vi "Configure FP for custom mode.vi"(0 "reference in":refnum<class "SPWB.lvclass">, 5 "error in (no error)":errorcluster, 7 "Analysis Type":T1) -> (14 "reference out":refnum<class "SPWB.lvclass">, 19 "error out":errorcluster)   [LabVIEW 2022 SP3, in "SPWB.lvclass"]
uses:
  SPWB.lvclass
  controls/Analysis Type.ctl
panel:
  out "Control Labels":string[](array[string])
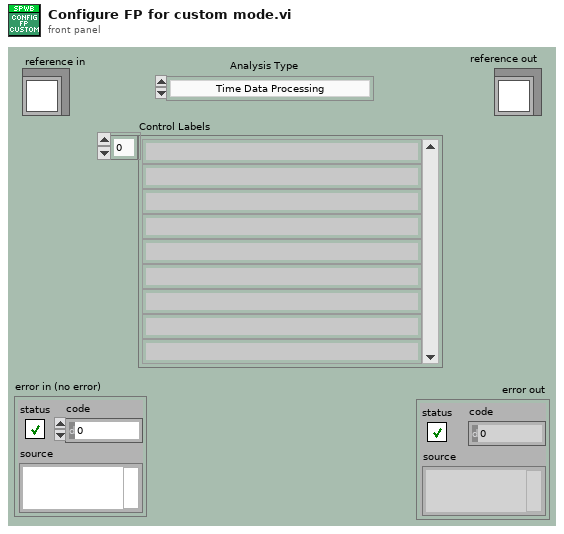
[diagram p1: front panel]
types:
  T1 = typedef "SPWB.lvclass/Analysis Type.ctl" = enum16{"Time Data Processing", "FFT Analysis", "Time Frequency Analysis", "Transfer Functions"}
  T2 = typedef "Generic Utilities.lvclass/FP Refnums.ctl" = cluster{"Panel refnum":refnum<vi>, "Control Labels":string[], "Refnums":refnum<vi>[]}
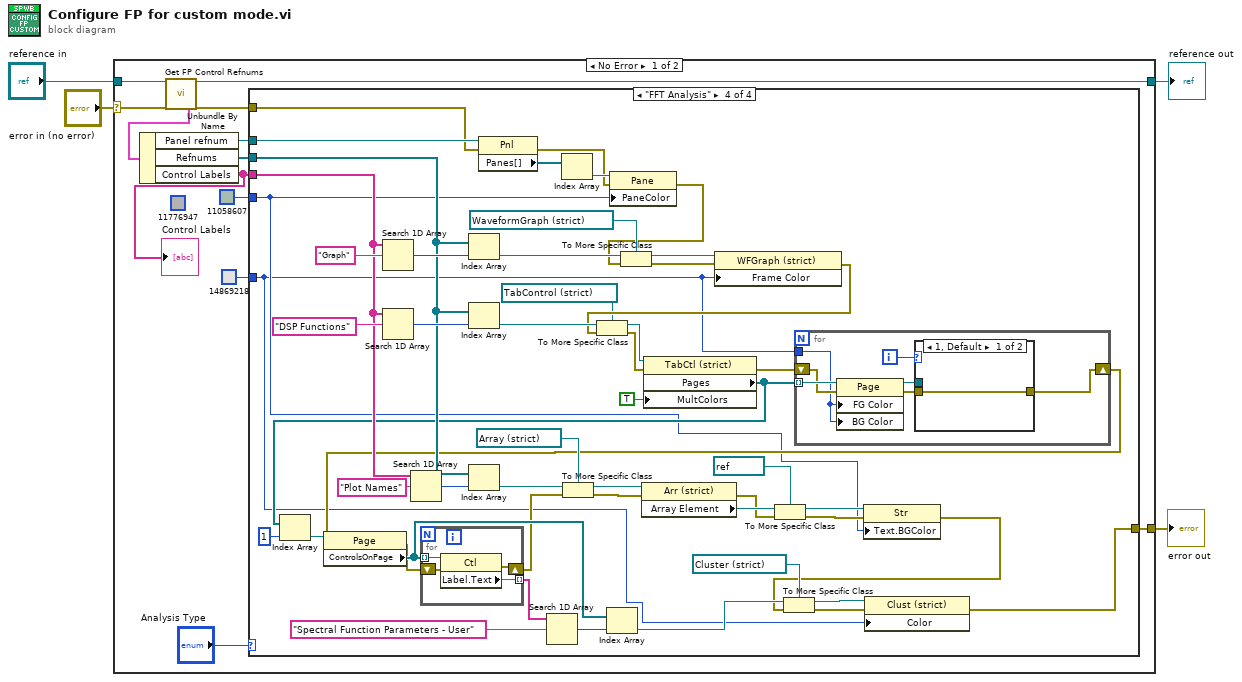
[diagram p0: block diagram]
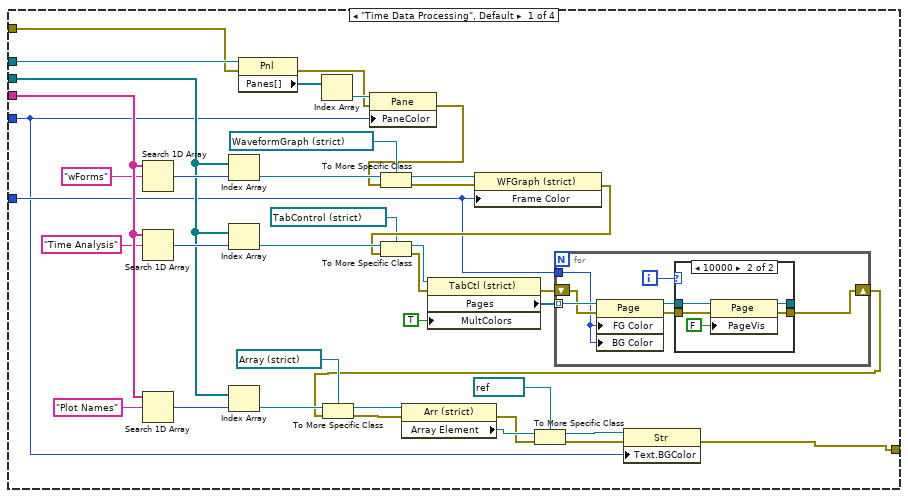
[diagram p2: hidden frame]
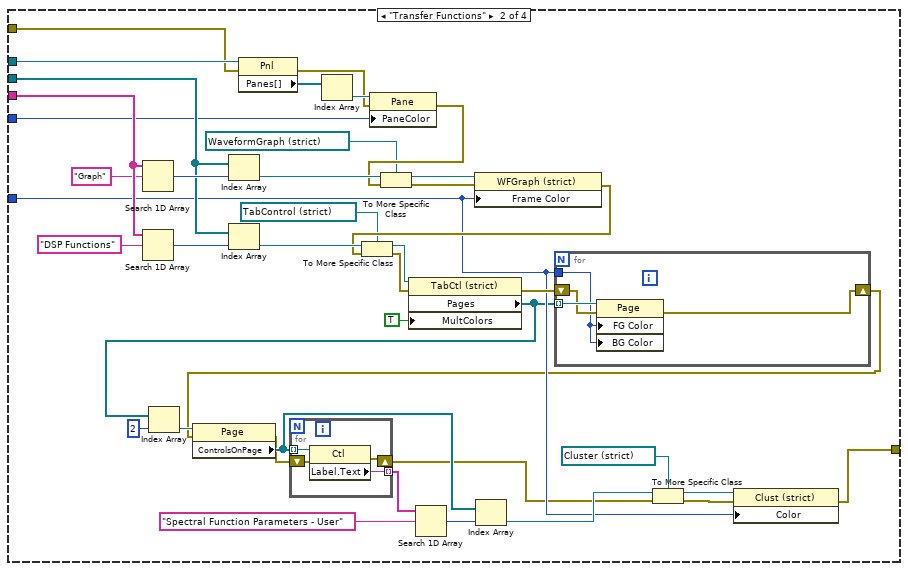
[diagram p4: hidden frame]
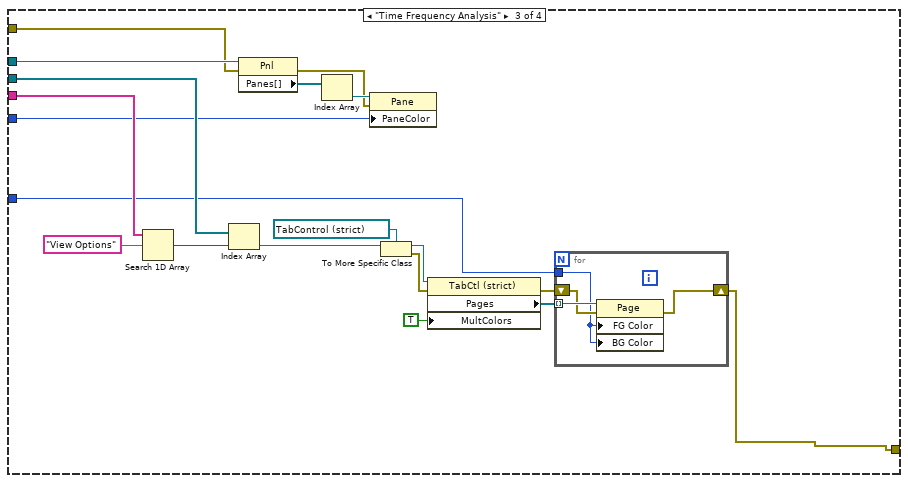
[diagram p5: hidden frame]
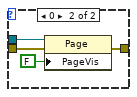
[diagram p6: hidden frame]
diagram:
  n1 = case shown="No Error" "error in (no error)" {
    selector: "error in (no error)" -> [w15 w210]
    tunnel: [w8 w210] -> w3
    tunnel: [w14 w209] -> w1
    tunnel: "reference in" -> [w16 w209]
    frame No Error {
      (unwired) u32 11776947
      n2 = call-dynamic "Get FP Control Refnums.vi"("reference in"=w16, "error in (no error)"=w15) -> ("FP Refnums"=w12:T2, "reference out"=w14:refnum<class "SPWB.lvclass">, "error out"=w9:errorcluster)  [unwired: 15 in]
      n3 = Unbundle By Name(w12) -> ("Panel refnum"=w10:refnum<vi>, "Refnums"=w11:refnum<vi>[], "Control Labels"=w7:string[])
      "Control Labels" <- w7
      n4 = case shown="\"FFT Analysis\"" "Analysis Type" {
        tunnel: w11 -> [w26 w94 w126 w157]
        tunnel: w10 -> [w25 w93 w125 w166]
        tunnel: w7 -> [w24 w92 w124 w155]
        tunnel: w9 -> [w20 w89 w122 w164]
        tunnel: [w18 w74 w118 w154] -> w8
        tunnel: u32 11058607 -> [w17 w88 w121 w142]
        tunnel: u32 14869218 -> [w19 w75 w120 w141]
        frame "Time Data Processing", Default {
          n5 = Search 1D Array(1D array=w24, element="wForms") -> (index of element=w52:i32)  [unwired: 1 in]
          n6 = Search 1D Array(1D array=w24, element="Time Analysis") -> (index of element=w47:i32)  [unwired: 1 in]
          n7 = Search 1D Array(1D array=w24, element="Plot Names") -> (index of element=w38:i32)  [unwired: 1 in]
          n8 = Index Array(array=w26, index=w52) -> (element=w51:refnum<vi>)
          n9 = Index Array(array=w26, index=w47) -> (element=w48:refnum<vi>)
          n10 = Index Array(array=w26, index=w38) -> (element=w35:refnum<vi>)
          n11 = property class="Pnl"(reference=w25, error in=w20) -> (error out=w53:errorcluster, "Panes[]"=w55:refnum<vi>[])  [unwired: 1 out]
          n12 = Index Array(array=w55) -> (element=w54:refnum<vi>)  [unwired: 1 in]
          n13 = property class="Pane"(reference=w54, error in=w53, "PaneColor"=w17) -> (error out=w45:errorcluster)  [unwired: 1 out]
          n14 = To More Specific Class(target class=refnum<vi> refnum ("wForms"), reference=w51, error in=w45) -> (specific class reference=w49:refnum<vi>, error out=w44:errorcluster)
          n15 = property class="WFGraph (strict)"(reference=w49, error in=w44, "Frame Color"=w19) -> (error out=w43:errorcluster)  [unwired: 1 out]
          n16 = To More Specific Class(target class=refnum<vi> refnum ("Time Analysis"), reference=w48, error in=w43) -> (specific class reference=w46:refnum<vi>, error out=w42:errorcluster)
          n17 = property class="TabCtl (strict)"(reference=w46, error in=w42, "MultColors"=TRUE ("Allow Multiple Colors")) -> (error out=w41:errorcluster, "Pages"=w40:refnum<vi>[])  [unwired: 1 out]
          n18 = for {
            shift-right: [w56] -> w28
            shift-left: w41 -> [w61]
            tunnel: w40 -> [w62] mode=indexing
            tunnel: w19 -> [w60]
            i -> [w57]
            n19 = property class="Page"(reference=w62, error in=w61, "FG Color"=w60, "BG Color"=w60) -> (reference out=w59:refnum<vi>, error out=w58:errorcluster)
            n20 = case shown="10000" w57 {
              tunnel: w59 -> [w64 w69]
              tunnel: [w64 w68] -> _
              tunnel: w58 -> [w63 w67]
              tunnel: [w63 w66] -> w56
              frame 0, Default {
              }
              frame 10000 {
                n21 = property class="Page"(reference=w69, error in=w67, "PageVis"=FALSE ("Page Visible")) -> (reference out=w68:refnum<vi>, error out=w66:errorcluster)
              }
            }
          }
          n22 = To More Specific Class(target class=refnum<vi> refnum ("Plot Names"), reference=w35, error in=w28) -> (specific class reference=w36:refnum<vi>, error out=w37:errorcluster)
          n23 = property class="Arr (strict)"(reference=w36, error in=w37) -> (error out=w29:errorcluster, "Array Element"=w32:refnum<vi>)  [unwired: 1 out]
          n24 = To More Specific Class(target class=refnum<vi> refnum ("String"), reference=w32, error in=w29) -> (specific class reference=w30:refnum<vi>, error out=w33:errorcluster)
          n25 = property class="Str"(reference=w30, error in=w33, "Text.BGColor"=w17) -> (error out=w18:errorcluster)  [unwired: 1 out]
        }
        frame "Transfer Functions" {
          n26 = Search 1D Array(1D array=w92, element="Graph") -> (index of element=w106:i32)  [unwired: 1 in]
          n27 = Search 1D Array(1D array=w92, element="DSP Functions") -> (index of element=w102:i32)  [unwired: 1 in]
          n28 = Index Array(array=w94, index=w106) -> (element=w105:refnum<vi>)
          n29 = Index Array(array=w94, index=w102) -> (element=w103:refnum<vi>)
          n30 = property class="Pnl"(reference=w93, error in=w89) -> (error out=w107:errorcluster, "Panes[]"=w109:refnum<vi>[])  [unwired: 1 out]
          n31 = Index Array(array=w109) -> (element=w108:refnum<vi>)  [unwired: 1 in]
          n32 = property class="Pane"(reference=w108, error in=w107, "PaneColor"=w88) -> (error out=w100:errorcluster)  [unwired: 1 out]
          n33 = To More Specific Class(target class=refnum<vi> refnum ("Graph"), reference=w105, error in=w100) -> (specific class reference=w104:refnum<vi>, error out=w99:errorcluster)
          n34 = property class="WFGraph (strict)"(reference=w104, error in=w99, "Frame Color"=w75) -> (error out=w98:errorcluster)  [unwired: 1 out]
          n35 = To More Specific Class(target class=refnum<vi> refnum ("DSP Functions"), reference=w103, error in=w98) -> (specific class reference=w101:refnum<vi>, error out=w97:errorcluster)
          n36 = property class="TabCtl (strict)"(reference=w101, error in=w97, "MultColors"=TRUE ("Allow Multiple Colors")) -> (error out=w96:errorcluster, "Pages"=w73:refnum<vi>[])  [unwired: 1 out]
          n37 = Index Array(array=w73, index=2) -> (element=w80:refnum<vi>)
          n38 = for {
            shift-right: [w114] -> w72
            shift-left: w96 -> [w116]
            tunnel: w73 -> [w117] mode=indexing
            tunnel: w75 -> [w115]
            n39 = property class="Page"(reference=w117, error in=w116, "FG Color"=w115, "BG Color"=w115) -> (error out=w114:errorcluster)  [unwired: 1 out]
          }
          n40 = property class="Page"(reference=w80, error in=w72) -> (error out=w76:errorcluster, "ControlsOnPage"=w78:refnum<vi>[])  [unwired: 1 out]
          n41 = for {
            tunnel: w78 -> [w113] mode=indexing
            tunnel: [w112] -> w79 mode=indexing
            shift-right: [w110] -> w71
            shift-left: w76 -> [w111]
            n42 = property class="Ctl"(reference=w113, error in=w111) -> (error out=w110:errorcluster, "Label.Text"=w112:string)  [unwired: 1 out]
          }
          n43 = Search 1D Array(1D array=w79, element="Spectral Function Parameters - User") -> (index of element=w84:i32)  [unwired: 1 in]
          n44 = Index Array(array=w78, index=w84) -> (element=w77:refnum<vi>)
          n45 = To More Specific Class(target class=refnum<vi> refnum ("Spectral Function Parameters - User"), reference=w77, error in=w71) -> (specific class reference=w85:refnum<vi>, error out=w86:errorcluster)
          n46 = property class="Clust (strict)"(reference=w85, error in=w86, "Color"=w75) -> (error out=w74:errorcluster)  [unwired: 1 out]
        }
        frame "Time Frequency Analysis" {
          n47 = Search 1D Array(1D array=w124, element="View Options") -> (index of element=w132:i32)  [unwired: 1 in]
          n48 = Index Array(array=w126, index=w132) -> (element=w133:refnum<vi>)
          n49 = property class="Pnl"(reference=w125, error in=w122) -> (error out=w134:errorcluster, "Panes[]"=w136:refnum<vi>[])  [unwired: 1 out]
          n50 = Index Array(array=w136) -> (element=w135:refnum<vi>)  [unwired: 1 in]
          n51 = property class="Pane"(reference=w135, error in=w134, "PaneColor"=w121) -> ()  [unwired: 2 out]
          n52 = To More Specific Class(target class=refnum<vi> refnum ("View Options"), reference=w133) -> (specific class reference=w131:refnum<vi>, error out=w130:errorcluster)  [unwired: 1 in]
          n53 = property class="TabCtl (strict)"(reference=w131, error in=w130, "MultColors"=TRUE ("Allow Multiple Colors")) -> (error out=w129:errorcluster, "Pages"=w128:refnum<vi>[])  [unwired: 1 out]
          n54 = for {
            shift-right: [w137] -> w118
            shift-left: w129 -> [w139]
            tunnel: w128 -> [w140] mode=indexing
            tunnel: w120 -> [w138]
            n55 = property class="Page"(reference=w140, error in=w139, "FG Color"=w138, "BG Color"=w138) -> (error out=w137:errorcluster)  [unwired: 1 out]
          }
        }
        frame "FFT Analysis" {
          n56 = Search 1D Array(1D array=w155, element="Graph") -> (index of element=w189:i32)  [unwired: 1 in]
          n57 = Search 1D Array(1D array=w155, element="DSP Functions") -> (index of element=w184:i32)  [unwired: 1 in]
          n58 = Search 1D Array(1D array=w155, element="Plot Names") -> (index of element=w176:i32)  [unwired: 1 in]
          n59 = Index Array(array=w157, index=w189) -> (element=w188:refnum<vi>)
          n60 = Index Array(array=w157, index=w184) -> (element=w185:refnum<vi>)
          n61 = Index Array(array=w157, index=w176) -> (element=w173:refnum<vi>)
          n62 = property class="Pnl"(reference=w166, error in=w164) -> (error out=w190:errorcluster, "Panes[]"=w192:refnum<vi>[])  [unwired: 1 out]
          n63 = Index Array(array=w192) -> (element=w191:refnum<vi>)  [unwired: 1 in]
          n64 = property class="Pane"(reference=w191, error in=w190, "PaneColor"=w142) -> (error out=w182:errorcluster)  [unwired: 1 out]
          n65 = To More Specific Class(target class=refnum<vi> refnum ("wForms"), reference=w188, error in=w182) -> (specific class reference=w186:refnum<vi>, error out=w181:errorcluster)
          n66 = property class="WFGraph (strict)"(reference=w186, error in=w181, "Frame Color"=w141) -> (error out=w180:errorcluster)  [unwired: 1 out]
          n67 = To More Specific Class(target class=refnum<vi> refnum ("DSP Functions"), reference=w185, error in=w180) -> (specific class reference=w183:refnum<vi>, error out=w179:errorcluster)
          n68 = property class="TabCtl (strict)"(reference=w183, error in=w179, "MultColors"=TRUE ("Allow Multiple Colors")) -> (error out=w178:errorcluster, "Pages"=w152:refnum<vi>[])  [unwired: 1 out]
          n69 = Index Array(array=w152, index=1) -> (element=w150:refnum<vi>)
          n70 = for {
            shift-right: [w197] -> w145
            shift-left: w178 -> [w202]
            tunnel: w152 -> [w203] mode=indexing
            tunnel: w141 -> [w201]
            i -> [w198]
            n71 = property class="Page"(reference=w203, error in=w202, "FG Color"=w201, "BG Color"=w201) -> (reference out=w200:refnum<vi>, error out=w199:errorcluster)
            n72 = case shown="1, Default" w198 {
              tunnel: w200 -> [_ w208]
              tunnel: w199 -> [w204 w207]
              tunnel: [w204 w206] -> w197
              frame 1, Default {
              }
              frame 0 {
                n73 = property class="Page"(reference=w208, error in=w207, "PageVis"=FALSE ("Page Visible")) -> (error out=w206:errorcluster)  [unwired: 1 out]
              }
            }
          }
          n74 = property class="Page"(reference=w150, error in=w145) -> (error out=w144:errorcluster, "ControlsOnPage"=w148:refnum<vi>[])  [unwired: 1 out]
          n75 = for {
            tunnel: w148 -> [w196] mode=indexing
            tunnel: [w195] -> w149 mode=indexing
            shift-right: [w193] -> w143
            shift-left: w144 -> [w194]
            n76 = property class="Ctl"(reference=w196, error in=w194) -> (error out=w193:errorcluster, "Label.Text"=w195:string)  [unwired: 1 out]
          }
          n77 = Search 1D Array(1D array=w149, element="Spectral Function Parameters - User") -> (index of element=w158:i32)  [unwired: 1 in]
          n78 = To More Specific Class(target class=refnum<vi> refnum ("Plot Names"), reference=w173, error in=w143) -> (specific class reference=w174:refnum<vi>, error out=w175:errorcluster)
          n79 = Index Array(array=w148, index=w158) -> (element=w147:refnum<vi>)
          n80 = property class="Arr (strict)"(reference=w174, error in=w175) -> (error out=w167:errorcluster, "Array Element"=w170:refnum<vi>)  [unwired: 1 out]
          n81 = To More Specific Class(target class=refnum<vi> refnum ("String"), reference=w170, error in=w167) -> (specific class reference=w168:refnum<vi>, error out=w171:errorcluster)
          n82 = property class="Str"(reference=w168, error in=w171, "Text.BGColor"=w142) -> (error out=w146:errorcluster)  [unwired: 1 out]
          n83 = To More Specific Class(target class=refnum<vi> refnum ("Spectral Function Parameters - User"), reference=w147, error in=w146) -> (specific class reference=w159:refnum<vi>, error out=w160:errorcluster)
          n84 = property class="Clust (strict)"(reference=w159, error in=w160, "Color"=w141) -> (error out=w154:errorcluster)  [unwired: 1 out]
        }
      }
    }
    frame Error {
    }
  }
  "error out" <- w3
  "reference out" <- w1
